vi "Frames.Compile.vi"(8 "error in (no error)":errorcluster, 10 "GUID":string, 11 "Section Ref in":T4 format="%.0x") -> (0 "error out":errorcluster, 1 "Frame Settings Array":T1[](array[typedef]) {"Signals"."Byte Order" items=["Little Endian", "Big Endian"]; "Signals"."Data Type" items=["Signed", "Unsigned", "IEEE Float"]}, 2 "Frame Refs":T5[](array[typedef]) {"Signal Refs" format="%.0x"}, 3 "Section Ref out":T4 format="%.0x")   [LabVIEW 2015, in "Diagnostics Addon System Explorer.lvlib"]
uses:
  Diagnostics Addon System Explorer.lvlib
  <vilib>/NI Veristand/Custom Device API/Custom Device Item Ref.ctl
  Types/Frame.Ref.ctl
  Shared/Types/Frame.Compile.ctl
  Shared/Types/Type.ctl
  Shared/Types/Signal.ctl
  Types/FG.Action.ctl
  Signal.FG.vi
  <vilib>/NI Veristand/Custom Device API/NI VeriStand - Get Custom Device Channel Data.vi
  <vilib>/NI Veristand/Custom Device API/NI VeriStand - Get Item Description.vi
  <vilib>/NI Veristand/Custom Device API/NI VeriStand - Get Item Property.vi
  <vilib>/NI Veristand/Custom Device API/Get Item Property (String).vi
  <vilib>/NI Veristand/Custom Device API/Get Item Property (Double).vi
  <vilib>/NI Veristand/Custom Device API/Get Item Property (U32).vi
  <vilib>/NI Veristand/Custom Device API/NI VeriStand - Set Item Property.vi
  <vilib>/NI Veristand/Custom Device API/Set Item Property (String).vi
  <vilib>/NI Veristand/Custom Device API/Set Item Property (Double).vi
  <vilib>/NI Veristand/Custom Device API/Set Item Property (U32).vi
  Shared/SubVIs/GUID Lookup.vi
  <vilib>/NI Veristand/Custom Device Tools/Custom Device Utility Library/NI VeriStand - Search for Item by GUID.vi
  <vilib>/NI Veristand/Custom Device Tools/Custom Device Utility Library/Custom Device Utility Library.lvlib
  <vilib>/NI Veristand/Custom Device API/Custom Device API.lvlib
  Shared/Diagnostics Addon Shared.lvlib
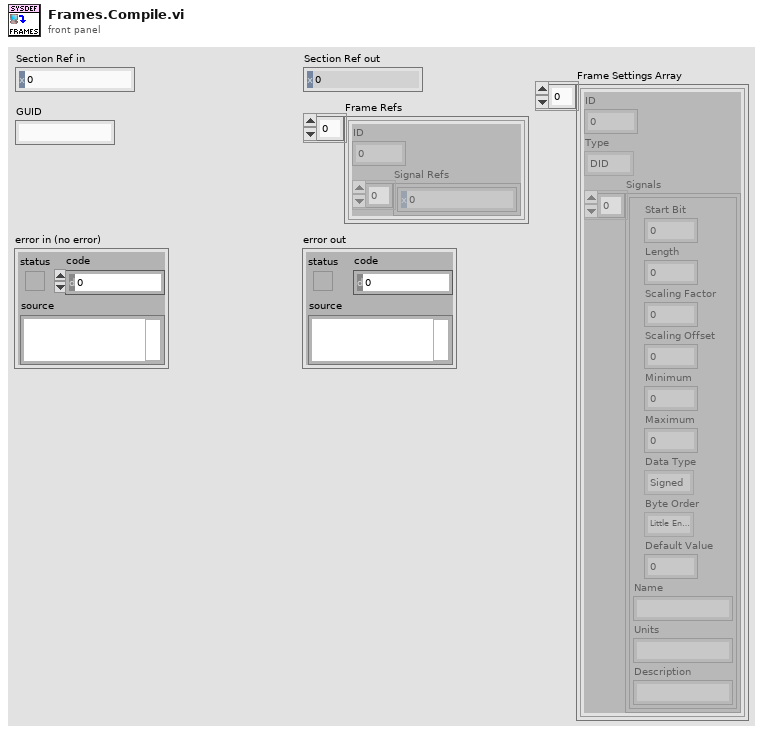
[diagram p1: front panel]
types:
  T1 = typedef "Diagnostics Addon Shared.lvlib/Frame.Compile.ctl" = cluster{"ID":u32, "Type":T2, "Signals":T3[]}
  T2 = typedef "Diagnostics Addon Shared.lvlib/Type.ctl" = enum16{"DID", "CDID", "PID", "CPID", "Read Memory", "Write Memory", "DTC Control", "IO Cmd", "IO Resp", "Routine Start Cmd", "Routine Start Resp", "Routine Request Cmd", "Routine Request Resp", "Routine Stop Cmd", "Routine Stop Resp"}
  T3 = typedef "Diagnostics Addon Shared.lvlib/Signal.ctl" = cluster{"Start Bit":u8, "Length":u8, "Scaling Factor":dbl, "Scaling Offset":dbl, "Minimum":dbl, "Maximum":dbl, "Data Type":u32, "Byte Order":u32, "Default Value":dbl, "Name":string, "Units":string, "Description":string}
  T4 = typedef "Custom Device API.lvlib/Custom Device Item Ref.ctl" = u64
  T5 = typedef "Diagnostics Addon System Explorer.lvlib/Frame.Ref.ctl" = cluster{"ID":u32, "Signal Refs":T4[]}
  T6 = typedef "Diagnostics Addon System Explorer.lvlib/FG.Action.ctl" = enum16{"Get", "Set"}
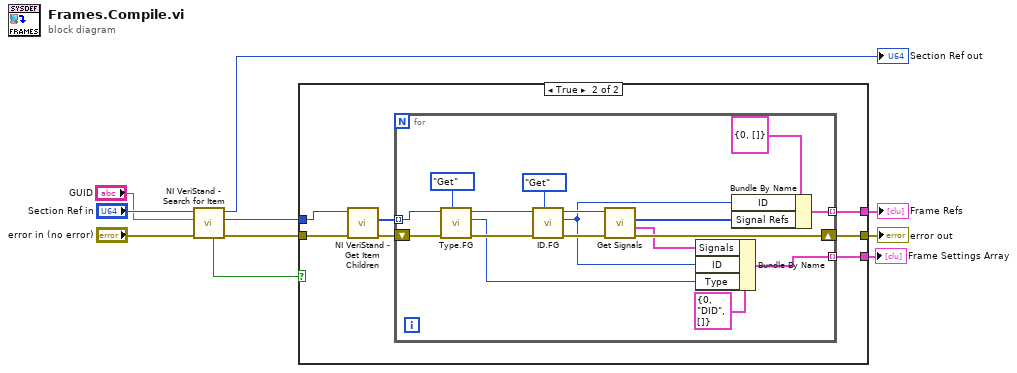
[diagram p0: block diagram]
diagram:
  n1 = call-poly <vilib>:"NI VeriStand - Search for Item.vi"("error in"="error in (no error)", "Item GUID"="GUID", "Section Ref in"="Section Ref in") -> ("error out"=w4:errorcluster, "Item Ref"=w5:T4, "Section Ref out"=→"Section Ref out":T4, "Found"=w2:bool)  [unwired: 5 in]
  n2 = case shown="True" w2 {
    tunnel: [w11 w18] -> w9
    tunnel: [_ w17] -> w8
    tunnel: w5 -> [_ w14]
    tunnel: w4 -> [w11 w13]
    tunnel: [_ w12] -> w1
    frame False {
    }
    frame True {
      n3 = call <vilib>:"NI VeriStand - Get Item Children.vi"("error in (no error)"=w13, "Item Ref in"=w14) -> ("error out"=w15:errorcluster, "Child Refs"=w16:T4[])  [unwired: 6 in, 2 out]
      n4 = for {
        shift-right: [w28] -> w18
        shift-left: w15 -> [w22]
        tunnel: w16 -> [w35] mode=indexing
        tunnel: [w33] -> w17 mode=indexing
        tunnel: [w24] -> w12 mode=indexing
        n5 = call "Type.FG.vi"("Action"=FG.Action."Get", "error in (no error)"=w22, "Device Item Ref in"=w35) -> ("error out"=w21:errorcluster, "Type"=w19:T2, "Device Item Ref out"=w23:T4)  [unwired: 6 in]
        n6 = call "ID.FG.vi"("Action"=FG.Action."Get", "error in (no error)"=w21, "Device Item Ref in"=w23) -> ("error out"=w30:errorcluster, "ID"=w26:u32, "Device Item Ref out"=w31:T4)  [unwired: 6 in]
        n7 = call "Get Signals.vi"("error in (no error)"=w30, "Device Item Ref out"=w31) -> ("error out"=w28:errorcluster, "Parameters"=w25:T3[], "Child Refs"=w29:T4[])  [unwired: 6 in, 1 out]
        n8 = Bundle By Name(cluster=T1 {"ID"=0, "Type"=enum."DID", "Signals"=[]} ("PID In"), "Signals"=w25, "ID"=w26, "Type"=w19) -> (w24:T1)
        n9 = Bundle By Name(cluster=T5 {"ID"=0, "Signal Refs"=[]}, "ID"=w26, "Signal Refs"=w29) -> (w33:T5)
      }
    }
  }
  "error out" <- w9
  "Frame Refs" <- w8
  "Frame Settings Array" <- w1
